vi "IKA_Eurostar60_Test.vi"() -> ()   [LabVIEW 2017]
uses:
  IKA_Eurostar60.ctl
panel:
  in  "Set_parametro":dbl format="%.3f"
  out "Read_parametro":dbl format="%.3f"
  in  "Command":T1=enum."READ NOMBRE APARATO"
  in  "SEND":bool
  out "Read_string":string
  out "error out":errorcluster
  in  "VISA resource name":refnum<visa-resource-name>="COM42"
  in  "stop":bool
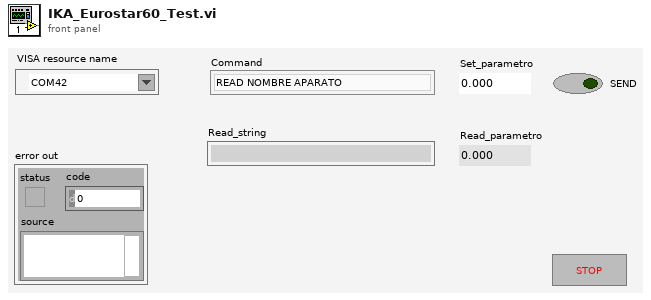
[diagram p1: front panel]
types:
  T1 = typedef "IKA_Eurostar60.ctl" = enum16{"INICIALIZAR", "READ NOMBRE APARATO", "READ VALOR PT100", "READ VELOCIDAD ACTUAL", "READ PAR DE GIRO ACTUAL", "READ VELOCIDAD NOMINAL", "READ LIMITE PAR DE GIRO", "READ LIMITE VELOCIDAD", "READ VELOCIDAD SEGURIDAD", "SET VELOCIDAD NOMINAL", "SET LIMITE PAR DE GIRO", "SET LIMITE VELOCIDAD", "SET VELOCIDAD SEGURIDAD", "ARRANCAR MOTOR", "DETENER MOTOR", "RESET", "SET SENTIDO DE GIRO", "READ SENTIDO DE GIRO", "FINALIZAR"}
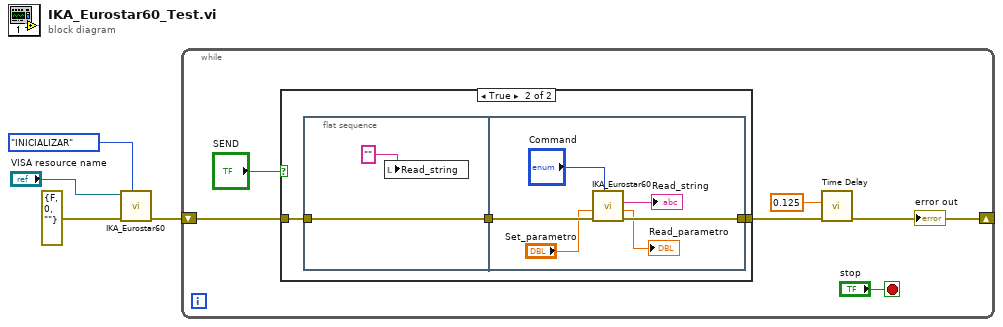
[diagram p0: block diagram]
diagram:
  n1 = call "IKA_Eurostar60.vi"("Command"=IKA_Eurostar60."INICIALIZAR", "Error in"=errorcluster {"status"=FALSE, "code"=0, "source"=""} ("error in (no error)"), "VISA Paar mPDS2000"="VISA resource name") -> ("error out"=w2:errorcluster)  [unwired: 6 in, 2 out]
  n2 = while {
    shift-right: [w6] -> _
    shift-left: w2 -> [w9]
    stop <- "stop" stop-if-true
    n3 = case shown="True" "SEND" {
      tunnel: w9 -> [w11 w14]
      tunnel: [w11 w13] -> w5
      frame False {
      }
      frame True {
        n4 = flat-sequence {
          tunnel: w14 -> [w16]
          tunnel: [w16] -> w12
          tunnel: [w19] -> w13
          tunnel: w12 -> [w22]
          frame #0 {
            n5 = local write "Read_string"("" ("Read_string")) -> ()
          }
          frame #1 {
            n6 = call "IKA_Eurostar60.vi"("Command"="Command", "Error in"=w22, "Set_parametro"="Set_parametro") -> ("error out"=w19:errorcluster, "Read_parametro"=→"Read_parametro":dbl, "read string"=→"Read_string":string)  [unwired: 6 in]
          }
        }
      }
    }
    n7 = call "Time Delay"("error in (no error)"=w5, "Delay Time (s)"=0.125) -> ("error out"=w6:errorcluster)  [unwired: 9 in]
    "error out" <- w6
  }
